vi "check if a string a whole number.vi"(11 "input string":string="0x014b4f5354414c5f") -> (3 "is a whole number?":bool=TRUE)   [LabVIEW 2010]
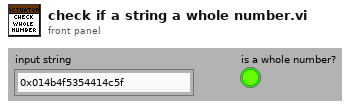
[diagram p1: front panel]
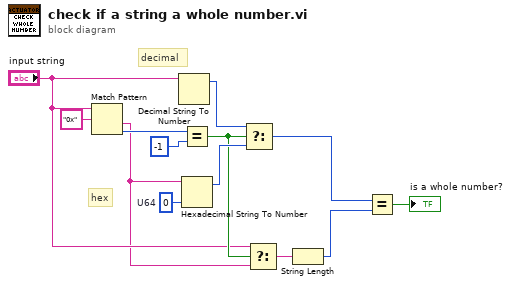
[diagram p0: block diagram]
diagram:
  w3 = u64 0  # U64
  # "hex"
  # "decimal"
  n1 = Match Pattern(string="input string", regular expression="0x") -> (after substring=w1:string, offset past match=w12:i32)  [unwired: 1 in, 2 out]
  n2 = Decimal String To Number(string="input string") -> (offset past number=w10:i32)  [unwired: 2 in, 1 out]
  n3 = Equal?(x=w12, y=-1) -> (x = y?=w8:bool)
  n4 = Hexadecimal String To Number(string=w1, default (0uL)=w3) -> (offset past number=w9:i32)  [unwired: 1 in, 1 out]
  n5 = Select(t=w10, s=w8, f=w9) -> (s? t:f=w4:i32)
  n6 = Select(t="input string", s=w8, f=w1) -> (s? t:f=w6:string)
  n7 = String Length(string=w6) -> (length=w5:i32)
  n8 = Equal?(x=w4, y=w5) -> (x = y?=→"is a whole number?":bool)
